vi "MPI_check.vi"() -> ()   [LabVIEW 2012]
uses:
  Instance           2 17Saved   MPI_check .vi
  <vilib>/express/express shared/transition.llb/Dynamic To Waveform Array.vi
  <vilib>/express/express shared/transition.llb/Waveform Array To Dynamic.vi
  <vilib>/express/express arith-compare/Formula/Block/exnFormulaBlock how many pts in the wave.vi
  <vilib>/express/express shared/ex_Modify Signal Name.vi
  Instance           5 17Saved   MPI_check .vi
  Instance           4 17Saved   MPI_check .vi
  Instance           6 17Saved   MPI_check .vi
  <vilib>/express/express arith-compare/Formula/XNode/ExpressFormulaBlockNode.xnode
panel:
  in  "Pol0 /Pol1":bool
  out "max":dbl
  out "min":dbl
  out "XYグラフ":cluster{"データ2":dbl[], "Array":dbl[]}[](graph)=[{"データ2"=[22.005, 22.01, 22.015, 22.02, 22.025, 22.03, 22.035, 22.04, 22.045, 22.05, 22.055, 22.06, 22.065, 22.07, 22.075, 22.08, 22.085, 22.09, 22.095, 22.1, 22.105, 22.11, 22.115, 22.12, 22.125, 22.13, 22.135, 22.14, 22.145, 22.15, 22.155, 22.16, 22.165, 22.17, 22.175, 22.18, 22.185, 22.19, 22.195, 22.2, 22.205, 22.21, 22.215, 22.22, 22.225, 22.23, 22.235, 22.24, 22.245, 22.25, 22.255, 22.26, 22.265, 22.27, 22.275, 22.28, 22.285, 22.29, 22.295, 22.3, 22.305, 22.31, 22.315, 22.32, 22.325, 22.33, 22.335, 22.34, 22.345, 22.35, 22.355, 22.36, 22.365, 22.37, 22.375, 22.38, 22.385, 22.39, 22.395, 22.4, 22.405, 22.41, 22.415, 22.42, 22.425, 22.43, 22.435, 22.44, 22.445, 22.45, 22.455, 22.46, 22.465, 22.47, 22.475, 22.48, 22.485, 22.49, 22.495, 22.5, 22.505, 22.51, 22.515, 22.52, 22.525, 22.53, 22.535, 22.54, 22.545, 22.55, 22.555, 22.56, 22.565, 22.57, 22.575, 22.58, 22.585, 22.59, 22.595, 22.6, 22.605, 22.61, 22.615, 22.62, 22.625, 22.63, 22.635, 22.64, 22.645, 22.65, 22.655, 22.66, 22.665, 22.67, 22.675, 22.68, 22.685, 22.69, 22.695, 22.7, 22.705, 22.71, 22.715, 22.72, 22.725, 22.73, 22.735, 22.74, 22.745, 22.75, 22.755, 22.76, 22.765, 22.77, 22.775, 22.78, 22.785, 22.79, 22.795, 22.8, 22.805, 22.81, 22.815, 22.82, 22.825, 22.83, 22.835, 22.84, 22.845, 22.85, 22.855, 22.86, 22.865, 22.87, 22.875, 22.88, 22.885, 22.89, 22.895, 22.9, 22.905, 22.91, 22.915, 22.92, 22.925, 22.93, 22.935, 22.94, 22.945, 22.95, 22.955, 22.96, 22.965, 22.97, 22.975, 22.98, 22.985, 22.99, 22.995, 23.0, 23.005, 23.01, 23.015, 23.02, 23.025, 23.03, 23.035, 23.04, 23.045, 23.05, 23.055, 23.06, 23.065, 23.07, 23.075, 23.08, 23.085, 23.09, 23.095, 23.1, 23.105, 23.11, 23.115, 23.12, 23.125, 23.13, 23.135, 23.14, 23.145, 23.15, 23.155, 23.16, 23.165, 23.17, 23.175, 23.18, 23.185, 23.19, 23.195, 23.2, 23.205, 23.21, 23.215, 23.22, 23.225, 23.23, 23.235, 23.24, 23.245, 23.25, 23.255, 23.26, 23.265, 23.27, 23.275, 23.28, 23.285, 23.29, 23.295, 23.3, 23.305, 23.31, 23.315, 23.32, 23.325, 23.33, 23.335, 23.34, 23.345, 23.35, 23.355, 23.36, 23.365, 23.37, 23.375, 23.38, 23.385, 23.39, 23.395, 23.4, 23.405, 23.41, 23.415, 23.42, 23.425, 23.43, 23.435, 23.44, 23.445, 23.45, 23.455, 23.46, 23.465, 23.47, 23.475, 23.48, 23.485, 23.49, 23.495, 23.5, 23.505, 23.51, 23.515, 23.52, 23.525, 23.53, 23.535, 23.54, 23.545, 23.55, 23.555, 23.56, 23.565, 23.57, 23.575, 23.58, 23.585, 23.59, 23.595, 23.6, 23.605, 23.61, 23.615, 23.62, 23.625, 23.63, 23.635, 23.64, 23.645, 23.65, 23.655, 23.66, 23.665, 23.67, 23.675, 23.68, 23.685, 23.69, 23.695, 23.7, 23.705, 23.71, 23.715, 23.72, 23.725, 23.73, 23.735, 23.74, 23.745, 23.75, 23.755, 23.76, 23.765, 23.77, 23.775, 23.78, 23.785, 23.79, 23.795, 23.8, 23.805, 23.81, 23.815, 23.82, 23.825, 23.83, 23.835, 23.84, 23.845, 23.85, 23.855, 23.86, 23.865, 23.87, 23.875, 23.88, 23.885, 23.89, 23.895, 23.9, 23.905, 23.91, 23.915, 23.92, 23.925, 23.93, 23.935, 23.94, 23.945, 23.95, 23.955, 23.96, 23.965, 23.97, 23.975, 23.98, 23.985, 23.99, 23.995, 24.0], "Array"=[0.9680299251292411, 0.9294486212237192, 0.8772742171761139, 0.813158160596254, 0.7391298816295282, 0.6575325565247022, 0.5709489403698398, 0.4821196165708932, 0.39385625067818447, 0.3089525942890383, 0.23009605597031144, 0.15978263819878863, 0.10023793277253462, 0.053346675382447896, 0.020593089113600912, 0.003013905151430624, 0.0011655477017831855, 0.0151065218026792, 0.04439556149663352, 0.08810559697847098, 0.14485309862396514, 0.21284186908947972, 0.2899198973548305, 0.37364747514023494, 0.4613744196454764, 0.5503239583234733, 0.6376806205286973, 0.720679354055124, 0.7966930458077087, 0.8633156763627082, 0.91843847637242, 0.9603166742771084, 0.9876247225962654, 0.9994982547511168, 0.9955614443828101, 0.975938901176738, 0.9412517266609081, 0.892597854822115, 0.8315172998076876, 0.7599434107076007, 0.680141676323111, 0.5946380169002408, 0.5061388325708421, 0.417445339162855, 0.3313649028622202, 0.25062218020090854, 0.17777287600742128, 0.11512284909290804, 0.06465512617501101, 0.027967134227981336, 0.006220138008264905, 0.00010248318236498618, 0.00980780850140868, 0.03502891666062452, 0.07496749784607903, 0.1283593981945642, 0.19351463335782734, 0.26837088064446324, 0.3505587565815338, 0.43747681370147906, 0.5263738827230985, 0.6144361537938718, 0.6988762404600475, 0.7770214072711258, 0.8463981684000217, 0.9048105795242858, 0.9504097448396196, 0.9817523391380176, 0.9978462925840207, 0.9981821921534284, 0.9827494058025943, 0.9520364189986349, 0.9070153729585829, 0.8491112940000488, 0.7801569879700094, 0.7023350274528384, 0.618108668005217, 0.5301438800879782, 0.44122496457442767, 0.3541664228120352, 0.2717238707648376, 0.19650681702272207, 0.13089606546618843, 0.0769683569955821, 0.03643063559786773, 0.01056601939065247, 0.00019318679288192212, 0.005640463348741297, 0.026735429420421855, 0.06281037769176004, 0.11272344773932204, 0.17489476871009993, 0.2473564661013127, 0.3278149498059953, 0.4137235118544341, 0.5023629359554848, 0.5909275673491313, 0.6766141186475786, 0.7567104007435727, 0.8286811702348003, 0.8902483760841304, 0.9394632655113541, 0.9747680667891093, 0.9950452965316512, 0.9996531307794346, 0.9884457202986314, 0.9617778070664585, 0.9204934958191519, 0.8658995360706926, 0.7997239602919581, 0.724061387452603, 0.6413067232032353, 0.5540793552488051, 0.4651402433157896, 0.3773045280177142, 0.29335242476357937, 0.2159412231341497, 0.14752117716195243, 0.09025794879265318, 0.045964059383183466, 0.016041518963841126, 0.0014374491885547087, 0.002614104616139885, 0.019534241221905602, 0.05166229526214906, 0.09798133517776363, 0.1570252499675188, 0.226925155190086, 0.3054685477318438, 0.3901693369464221, 0.4783465355096535, 0.567209119231127, 0.653944369802553, 0.7358069042174976, 0.8102055728640051, 0.8747854757532394, 0.9275025008686351, 0.9666880253152442, 0.9911017313190111, 0.9999708653207569, 0.9930146975178897, 0.9704534076498883, 0.9330011157706267, 0.8818432786004248, 0.8185991669188826, 0.7452706116809454, 0.6641786411664744, 0.5778900147535365, 0.4891359787006163, 0.40072581551675907, 0.31545792329272304, 0.2360312395511897, 0.16495981326739123, 0.10449322906437247, 0.05654540235297022, 0.022633999223761584, 0.0038323986001711653, 0.0007357171677934473, 0.013441972474582885, 0.041548980435440024, 0.08416708544309634, 0.13994732014591593, 0.20712410356687072, 0.28357112606336715, 0.36686865223287746, 0.454380111461703, 0.5433355518392694, 0.6309193159166231, 0.714359163157733, 0.7910140181386373, 0.8584575670497547, 0.914555056467845, 0.9575308635274579, 0.9860246987313817, 0.9991346624431167, 0.9964457922183215, 0.978043197381885, 0.9445093651095368, 0.896905723282741, 0.8367390436979394, 0.7659137490505888, 0.6866716332950753, 0.6015209033778958, 0.5131567883478997, 0.42437622875923836, 0.33798934665560465, 0.25673049832868455, 0.1831717252477731, 0.11964134265117474, 0.06815024266893596, 0.030328244664526403, 0.007372507462158419, 9.636339437649606e-06, 0.008472684191516134, 0.032493774836551, 0.07131258195251389, 0.12370039526664672, 0.18799901224339174, 0.26217322425395106, 0.34387523591131564, 0.43051897854192867, 0.5193619655896998, 0.6075920990288466, 0.6924166791507397, 0.7711508003458946, 0.841302334939208, 0.9006508151313546, 0.9473177162405876, 0.9798259166073142, 0.9971464521105524, 0.9987310854013794, 0.9845296589569947, 0.9549916826891028, 0.911052105854913, 0.8541017236242879, 0.7859431550080563, 0.7087337855534773, 0.624917480810663, 0.5371472320050633, 0.4482011823708686, 0.3608946921170164, 0.2779912253842638, 0.20211487984048757, 0.13566732756565839, 0.08075179625145272, 0.039106496895875476, 0.012049605170254505, 0.000437537932394422, 0.004637845536423225, 0.024517577964416726, 0.05944749301992984, 0.10832197338377517, 0.16959402210884963, 0.24132422886048885, 0.3212421570010009, 0.40681820846753086, 0.49534369174295195, 0.5840165585733068, 0.6700300956541448, 0.7506617639777549, 0.8233593738572199, 0.8858218679778136, 0.9360721554937775, 0.9725196917937285, 0.99401082313105, 0.9998653025890888, 0.989897821561387, 0.9644238752226364, 0.9242497763340614, 0.8706471334708149, 0.8053126014975356, 0.7303141782885572, 0.6480257475329702, 0.5610519395043299, 0.4721456881366298, 0.3841210939260605, 0.2997643507616988, 0.22174555606800606, 0.15253419568521212, 0.09432097859735329, 0.04894849562982796, 0.01785289693935595, 0.0020184343457974024, 0.0019463073526621375, 0.01763879895583135, 0.048599203381205214, 0.09384754803839764, 0.15195161205203445, 0.2210722595586952, 0.2990216528590923, 0.3833325028368308, 0.47133616469914075, 0.5602471071171343, 0.6472510811113946, 0.7295941979211472, 0.804670096325365, 0.8701024403555198, 0.9238201361460867, 0.9641228871256575, 0.9897350125655187, 0.9998458259976045, 0.9941352954257359, 0.972784173121773, 0.9364682743736631, 0.8863370862773226, 0.8239773836559786, 0.7513630037527185, 0.6707923694497573, 0.584815738557963, 0.4961544819138265, 0.40761494533085746, 0.3219996218846025, 0.24201844614660514, 0.17020301812099445, 0.10882647190726229, 0.05983152544153764, 0.024768988717918345, 0.004748676855992648, 0.0004042817354572913, 0.011873314096862991, 0.03879275099003439, 0.08031052633917292, 0.13511250091985771, 0.20146405808265766, 0.2772650086162801, 0.3601160668774083, 0.4473947940544698, 0.5363386047760449, 0.6241322097004485, 0.7079967263149675, 0.7852776373704022, 0.8535288128499507, 0.9105899359724091, 0.95465488250655, 0.9843288890246341, 0.9986727005790769, 0.9972323004208518, 0.9800532807410351, 0.947679399566344, 0.9011353694864381, 0.8418944229921307, 0.7718316810604164, 0.6931648009854195, 0.60838378209617, 0.5201721511826223, 0.4313220223031812, 0.3446457195398984, 0.26288676005695594, 0.1886330150659838, 0.1242347973674108, 0.07173046819672411, 0.03278191810164392, 0.008621964037795058, 1.5327694311269866e-05, 0.007234430180324381, 0.030050769229943066, 0.06774215185837222, 0.11911555353782287, 0.18254488034415858, 0.25602243881045345, 0.33722248433987134, 0.4235748367156198, 0.5123462325963059, 0.6007268399920246, 0.6859191963250605, 0.7652267549684179, 0.8361392375480118, 0.8964120903980675, 0.9441375301793481, 0.9778049298919268, 0.9963486339179164, 0.9991816886303289, 0.9862144209122592, 0.9578572765305661, 0.9150078285225689, 0.8590223668121428, 0.7916729683136282, 0.7150914063592507, 0.6317016748547125, 0.5441432629384004, 0.4551876086883927, 0.36765037632310354, 0.28430233353597417, 0.20778164991543258, 0.1405103924188862, 0.08461786102459615, 0.041873191174801296, 0.013629356308279616, 0.0007803429387812377, 0.00373285379354853, 0.022393434676345067, 0.05617143252155281, 0.10399769100960693, 0.1643583919818236, 0.23534297149073505, 0.31470459382630034, 0.39993126936622964, 0.4883253651966164, 0.5770889917977685, 0.6634125630964374, 0.7445637267429528, 0.8179738497516001, 0.8813193220229183, 0.9325951042912884, 0.970178192525905, 0.9928789899816455, 0.999978960848004, 0.9912533736664828, 0.9669784146314266, 0.9279224456208375, 0.8753216836620168, 0.8108410716363704, 0.7365215787616608, 0.6547155989197447, 0.5680124916317184, 0.4791566224905888, 0.39096049727174215, 0.30621573924044665, 0.22760472744156357, 0.15761569283659296]}, ...(2 in all)]
  in  "停止":bool
  in  "オフセット（mm）":dbl=23.053 step=0.001
  in  "周波数（GHｚ）":dbl=850.0
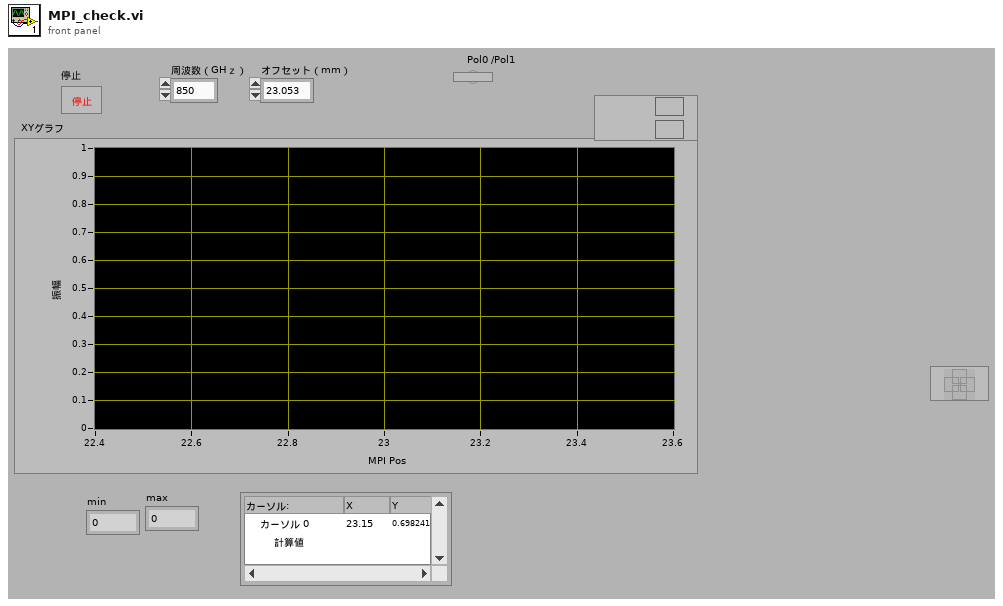
[diagram p1: front panel]
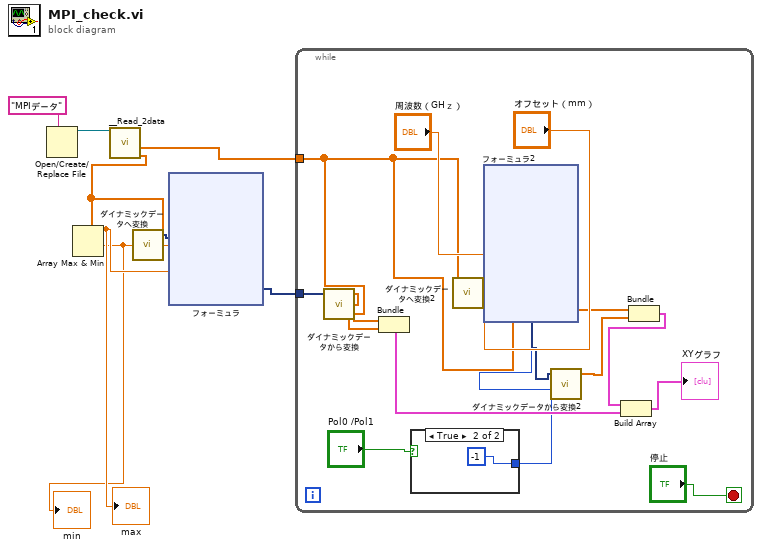
[diagram p0: block diagram]
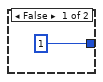
[diagram p2: hidden frame]
diagram:
  n1 = Open/Create/Replace File(prompt="MPIデータ") -> (refnum out=w8:refnum<file>)  [unwired: 5 in, 2 out]
  n2 = call "__Read_2data.vi"("refnum"=w8) -> ("データ2"=w5:dbl[], "データ1"=w3:dbl[])  [unwired: 3 in, 2 out]
  n3 = Array Max & Min(array=w5) -> (max value=w2:dbl, min value=w1:dbl)  [unwired: 2 out]
  "min" <- w1
  "max" <- w2
  n4 = call "ダイナミックデータへ変換"("Array"=w5) -> ("Dynamic Data Type"=w6:dynamicdata)  [unwired: 3 in]
  n5 = xnode "フォーミュラ"("X1"=w6, "min"=w1, "max"=w2) -> ("結果"=w4:dynamicdata)  [unwired: 1 in, 1 out]
  n6 = while {
    tunnel: w3 -> [w14]
    tunnel: w4 -> [w18]
    stop <- "停止" stop-if-true
    n7 = call "ダイナミックデータから変換"("Dynamic Data Type"=w18) -> ("Array"=w12:dbl[])  [unwired: 3 in]
    n8 = Bundle("データ1"=w14, "Array"=w12) -> (w13:cluster{"データ1":dbl[], "Array":dbl[]})  [unwired: 1 in]
    n9 = case shown="TRUE" "Pol0 /Pol1" {
      tunnel: [1 -1] -> w9
      frame False {
      }
      frame True {
      }
    }
    n10 = call "ダイナミックデータへ変換2"("Array"=w14) -> ("Dynamic Data Type"=w21:dynamicdata)  [unwired: 3 in]
    n11 = xnode "フォーミュラ2"("X1"=w21, "frq"="周波数（GHｚ）", "offset"="オフセット（mm）", "Pol"=w9) -> ("結果"=w17:dynamicdata)  [unwired: 1 in, 1 out]
    n12 = call "ダイナミックデータから変換2"("Dynamic Data Type"=w17) -> ("Array"=w15:dbl[])  [unwired: 3 in]
    n13 = Bundle("データ1"=w14, "Array"=w15) -> (w11:cluster{"データ1":dbl[], "Array":dbl[]})  [unwired: 1 in]
    n14 = Build Array(w11, w13) -> (→"XYグラフ":cluster{"データ1":dbl[], "Array":dbl[]}[])
  }
